vi "ARM CONTROL.vi"(8 "error in (no error)":errorcluster, 11 "control\ncluster":T1={"Axes"=[0.0, -0.007874015748031496, 0.0, 0.0, 0.015748031496062992, -0.007874015748031496], "Buttons"=[FALSE, FALSE, FALSE, FALSE, FALSE, FALSE, FALSE, FALSE, FALSE, FALSE], "POVs"=[-1]}) -> (0 "error out":errorcluster, 3 "control\ncluster out":T1={"Axes"=[0.0, -0.007874015748031496, 0.0, 0.0, 0.015748031496062992, -0.007874015748031496], "Buttons"=[FALSE, FALSE, FALSE, FALSE, FALSE, FALSE, FALSE, FALSE, FALSE, FALSE], "POVs"=[-1]})   [LabVIEW 2023]
uses:
  ctrl defs/ctrl controllers.ctl
  Global odometry.vi
panel:
  in  "notes":string="Joystick 1- co-pilot\n\nARM LOCK toggles pneumatic ratchet lock on both arms"
  in  "axis for\nRIGHT ARM":i32=5
  in  "axis for\nLEFT ARM":i32=1
  in  "button for\nARM LOCK":i32=4
  out "set\nLOCKs":bool
  out "Buttons":bool[](array[boolean])
  out "POVs":i16[](array[numeric])=[-1]
  out "Axes":dbl[](array[numeric])=[0.0, -0.007874015748031496, 0.0, 0.0, 0.015748031496062992, -0.007874015748031496]
  in  "axis scale":dbl=0.7 format="%#_13g"
  in  "axis dead band":dbl=0.025 format="%#_13g"
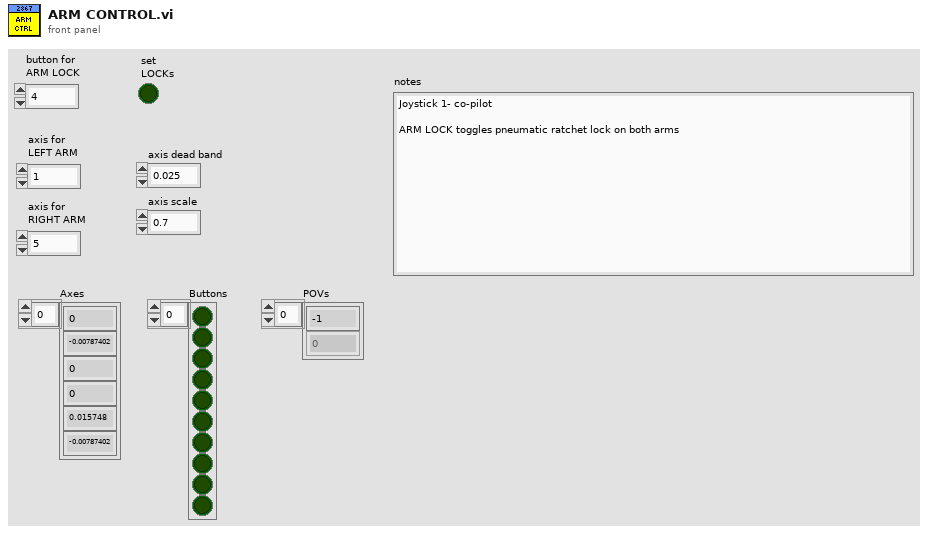
[diagram p1: front panel]
types:
  T1 = typedef "ctrl controllers.ctl" = cluster{"Axes":dbl[], "Buttons":bool[], "POVs":i16[]}
  T2 = cluster{"LEFT ARM":cluster{"VBus%":dbl, "LOCK?":bool, "LOCKED":bool}, "RIGHT ARM":cluster{"VBus%":dbl, "LOCK?":bool, "LOCKED":bool}}
  T3 = cluster{"VBus%":dbl, "LOCK?":bool, "LOCKED":bool}
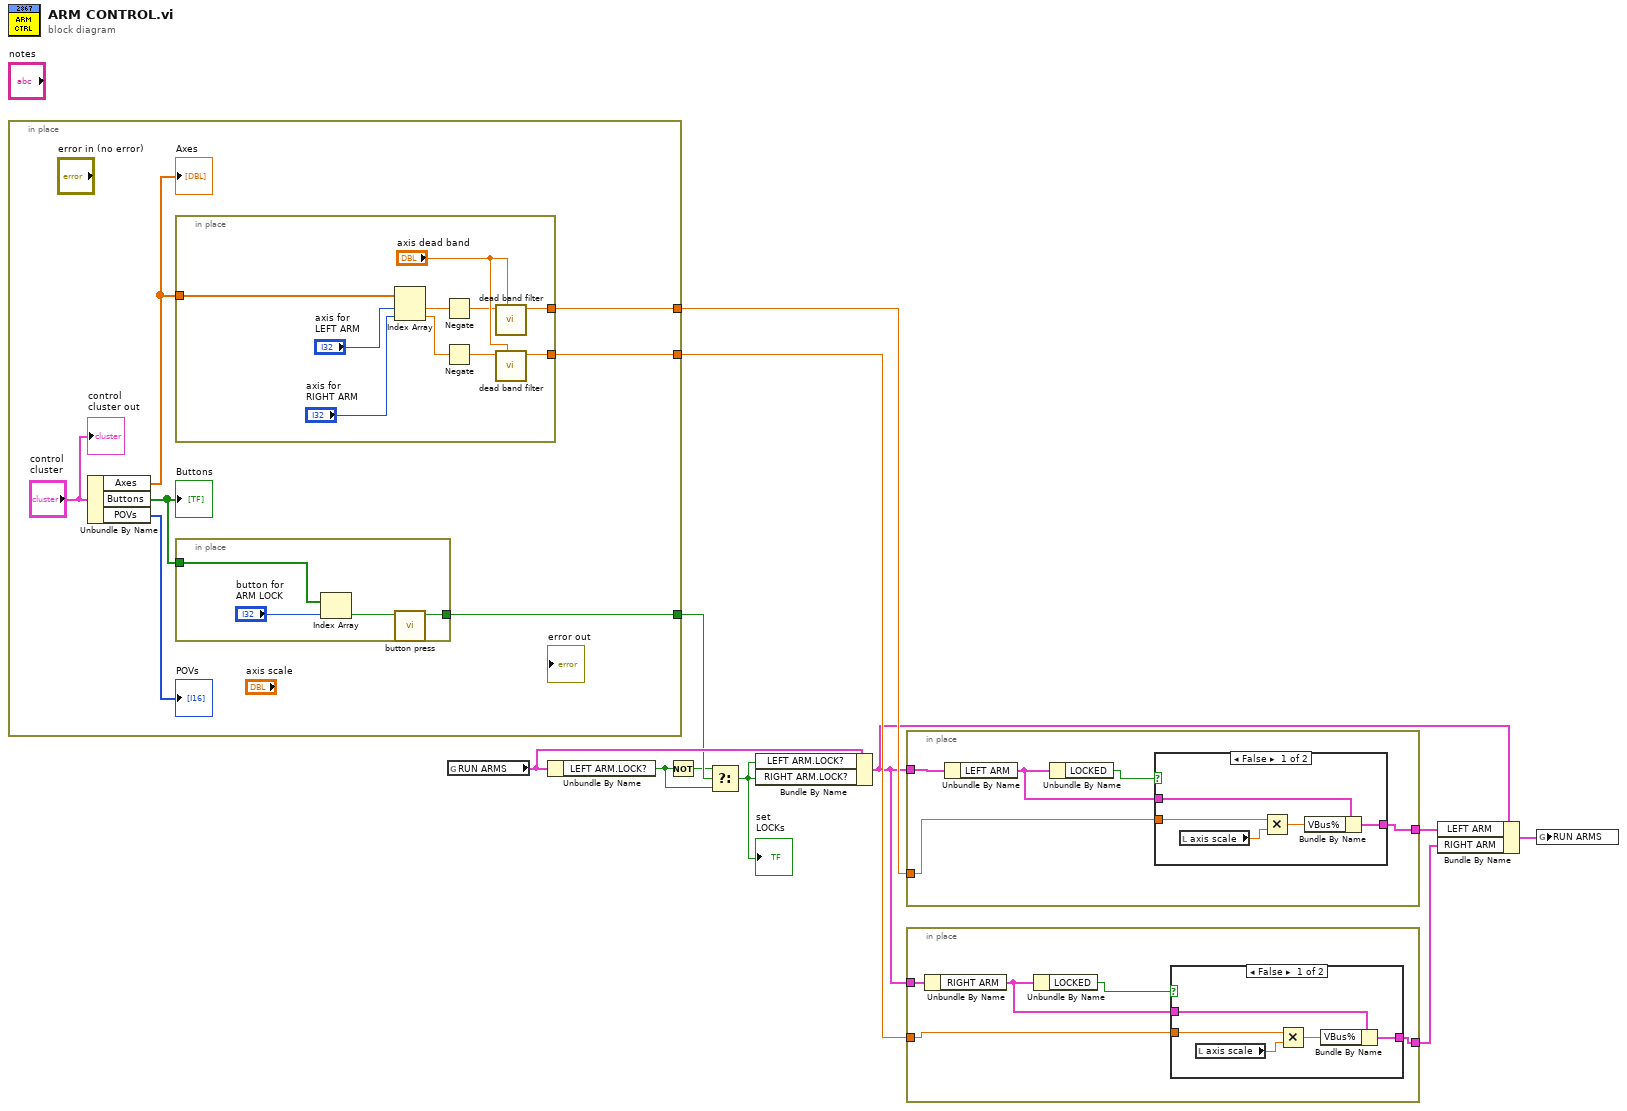
[diagram p0: block diagram]
diagram:
  n1 = in-place {
    in-place-border: [w18] -> w11
    in-place-border: [w17] -> w10
    in-place-border: [w12] -> w3
    n2 = Unbundle By Name("control\ncluster") -> ("Axes"=w15:dbl[], "Buttons"=w13:bool[], "POVs"=→"POVs":i16[])
    "Axes" <- w15
    "Buttons" <- w13
    n3 = in-place {
      in-place-border: [w21] -> w18
      in-place-border: [w20] -> w17
      in-place-border: w15 -> [w19]
      n4 = Index Array(array=w19, index #1="axis for\nLEFT ARM", index #2="axis for\nRIGHT ARM") -> (element #1=w25:dbl, element #2=w24:dbl)
      n5 = Negate(x=w25) -> (-x=w23:dbl)
      n6 = Negate(x=w24) -> (-x=w22:dbl)
      n7 = call "dead band filter.vi"("deadband"="axis dead band", "input"=w23) -> ("output"=w21:dbl)  [unwired: 9 in]
      n8 = call "dead band filter.vi"("deadband"="axis dead band", "input"=w22) -> ("output"=w20:dbl)  [unwired: 9 in]
    }
    n9 = in-place {
      in-place-border: w13 -> [w32]
      in-place-border: [w30] -> w12
      n10 = Index Array(array=w32, index="button for\nARM LOCK") -> (element=w31:bool)
      n11 = call "button press.vi"("button IN"=w31) -> ("Button Pressed?"=w30:bool)  [unwired: 10 in]
    }
    "control\ncluster out" <- "control\ncluster"
  }
  n12 = global read "Global odometry.vi" "RUN ARMS"() -> (w5:T2)
  n13 = Unbundle By Name(w5) -> ("LEFT ARM.LOCK?"=w4:bool)
  n14 = Not(x=w4) -> (.not. x?=w2:bool)
  n15 = Select(t=w2, s=w3, f=w4) -> (s? t:f=w1:bool)
  "set\nLOCKs" <- w1
  n16 = Bundle By Name(cluster=w5, "LEFT ARM.LOCK?"=w1, "RIGHT ARM.LOCK?"=w1) -> (w6:T2)
  n17 = in-place {
    in-place-border: w11 -> [w37]
    in-place-border: [w34] -> w8
    in-place-border: w6 -> [w33]
    n18 = Unbundle By Name(w33) -> ("LEFT ARM"=w35:T3)
    n19 = Unbundle By Name(w35) -> ("LOCKED"=w36:bool)
    n20 = case shown="False" w36 {
      tunnel: w37 -> [w42 _]
      tunnel: [w41 w43] -> w34
      tunnel: w35 -> [w40 w43]
      frame False {
        n21 = local read "axis scale"() -> (w38:dbl)
        n22 = Multiply(x=w42, y=w38) -> (x*y=w39:dbl)
        n23 = Bundle By Name(cluster=w40, "VBus%"=w39) -> (w41:T3)
      }
      frame True {
      }
    }
  }
  n24 = in-place {
    in-place-border: w10 -> [w46]
    in-place-border: [w45] -> w7
    in-place-border: w6 -> [w44]
    n25 = Unbundle By Name(w44) -> ("RIGHT ARM"=w48:T3)
    n26 = Unbundle By Name(w48) -> ("LOCKED"=w47:bool)
    n27 = case shown="False" w47 {
      tunnel: w46 -> [w52 _]
      tunnel: [w51 w54] -> w45
      tunnel: w48 -> [w50 w54]
      frame False {
        n28 = local read "axis scale"() -> (w49:dbl)
        n29 = Multiply(x=w52, y=w49) -> (x*y=w53:dbl)
        n30 = Bundle By Name(cluster=w50, "VBus%"=w53) -> (w51:T3)
      }
      frame True {
      }
    }
  }
  n31 = Bundle By Name(cluster=w6, "LEFT ARM"=w8, "RIGHT ARM"=w7) -> (w9:T2)
  n32 = global write "Global odometry.vi" "RUN ARMS"(w9) -> ()
